vi "Close Instrument.vi"(8 "error in (no error)":errorcluster, 11 "NI Sig Gen.lvclass in":refnum<class "NI Sig Gen.lvclass">) -> (0 "error out":errorcluster, 3 "NI Sig Gen.lvclass out":refnum<class "NI Sig Gen.lvclass">)   [LabVIEW 2011, in "NI Sig Gen.lvclass"]
uses:
  NI Sig Gen.lvclass
  NI Sig Gen.lvclass/NI Sig Gen.ctl
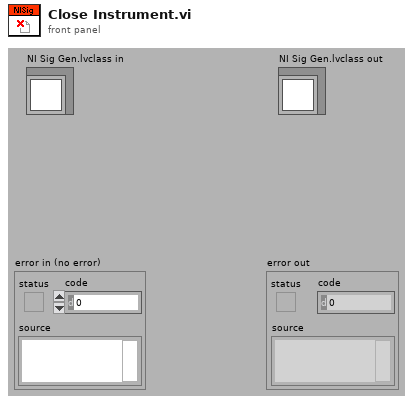
[diagram p1: front panel]
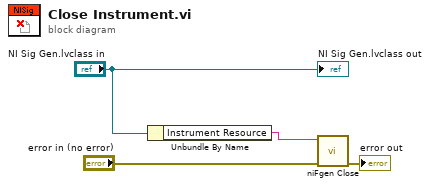
[diagram p0: block diagram]
diagram:
  n1 = Unbundle By Name("NI Sig Gen.lvclass in") -> ("Instrument Resource"=w1:string)
  n2 = call <instrlib>:"niFgen Close.vi"("error in (no error)"="error in (no error)", "Instrument Handle"=w1) -> ("error out"=→"error out":errorcluster)  [unwired: 9 out]
  "NI Sig Gen.lvclass out" <- "NI Sig Gen.lvclass in"
